vi "Configure Trigger Select.vi"(4 "Hold Type (0: TI)":u16(ring) items=["TI", "TL", "EV", "PS", "PL", "IS", "IL", "P2", "I2", "OFF"], 5 "QL (1: Channel 2)":u16(ring)=1 items=["Channel 1", "Channel 2", "Channel 3", "Channel 4", "Ext", "Ext10", "Line", "Pattern"], 6 "Trigger type":u16(ring) items=["Edge", "Dropout", "Glitch", "Interval", "Std", "Sng", "State Qualify", "Edge Qualify", "Width", "Logic", "Runt", "Slew"], 7 "Trigger Source (0: Channel 1)":u16(ring) items=["Channel 1", "Channel 2", "Channel 3", "Channel 4", "Ext", "Ext10", "Line", "Pattern"], 8 "error in (no error)":errorcluster, 9 "Hold Value 2 (6 ns)":dbl=6e-09, 10 "Hold Value 1 (4 ns)":dbl=4e-09, 11 "VISA resource name":refnum<visa-resource-name>) -> (0 "error out":errorcluster, 3 "VISA resource name out":refnum<visa-resource-name>)   [LabVIEW 2013, in "LeCroy Wave Series.lvlib"]
doc: "Selects the condition that will trigger the acquisition of waveforms. Depending on the trigger type, additional parameters may need to be specified."
uses:
  <instrlib>/LeCroy Wave Series/LeCroy Wave Series.lvlib
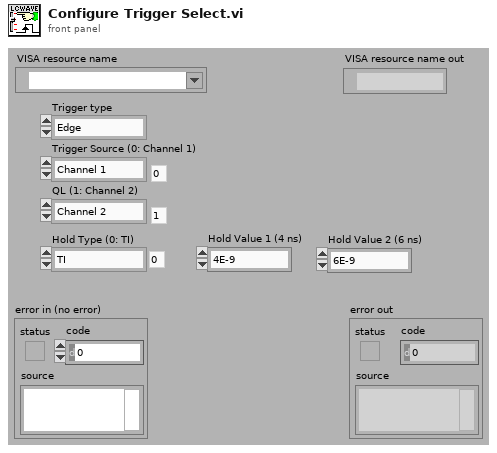
[diagram p1: front panel]
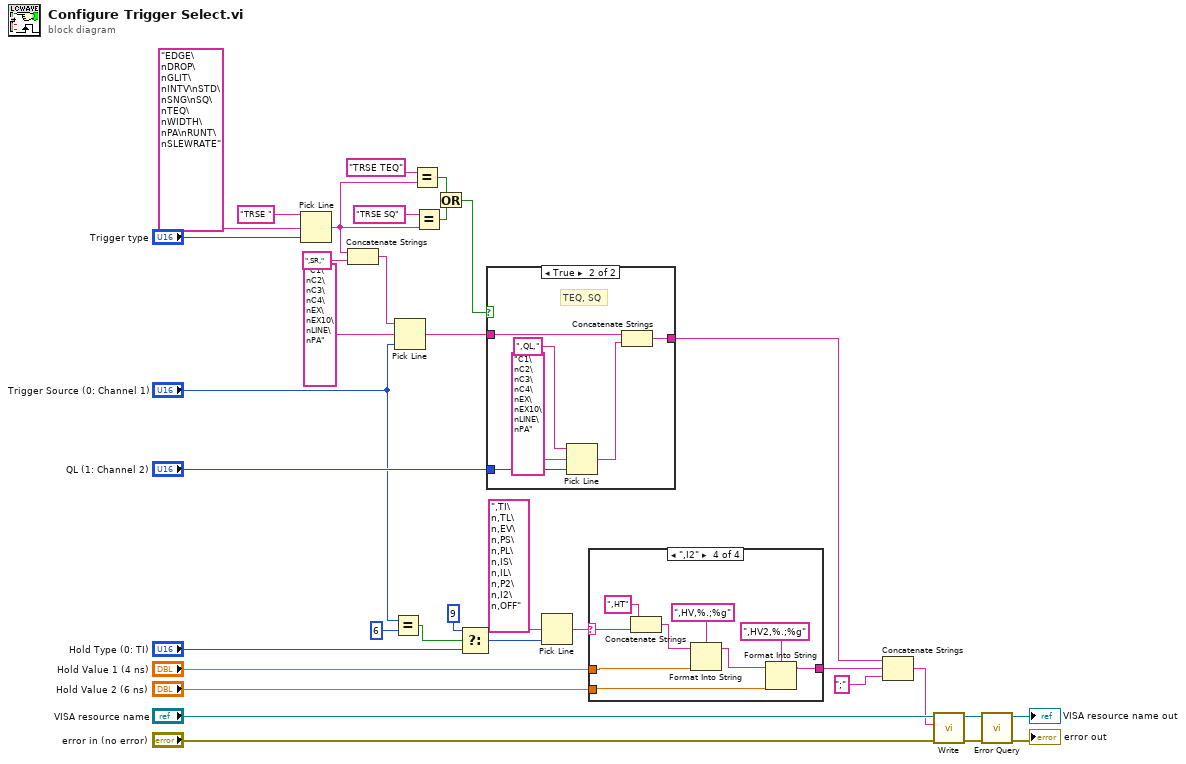
[diagram p0: block diagram]
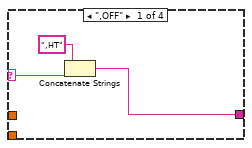
[diagram p2: hidden frame]
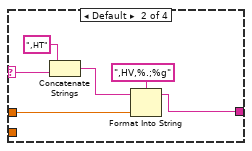
[diagram p3: hidden frame]
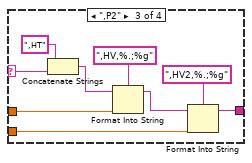
[diagram p4: hidden frame]
diagram:
  n1 = Pick Line(string ("")="TRSE ", multi-line string="EDGE\nDROP\nGLIT\nINTV\nSTD\nSNG\nSQ\nTEQ\nWIDTH\nPA\nRUNT\nSLEWRATE", line index="Trigger type") -> (output string=w25:string)
  n2 = Concatenate Strings(w25, ",SR,") -> (w27:string)
  n3 = Equal?(x="Trigger Source (0: Channel 1)", y=u16 6) -> (x = y?=w10:bool)
  n4 = Pick Line(string ("")=w27, multi-line string="C1\nC2\nC3\nC4\nEX\nEX10\nLINE\nPA", line index="Trigger Source (0: Channel 1)") -> (output string=w20:string)
  n5 = Equal?(x="TRSE TEQ", y=w25) -> (x = y?=w23:bool)
  n6 = Equal?(x="TRSE SQ", y=w25) -> (x = y?=w22:bool)
  n7 = Or(x=w23, y=w22) -> (x .or. y?=w21:bool)
  n8 = Select(t=u16 9, s=w10, f="Hold Type (0: TI)") -> (s? t:f=w5:u16)
  n9 = case shown="True" w21 {
    tunnel: w20 -> [w35 w37]
    tunnel: [w35 w38] -> w14
    tunnel: "QL (1: Channel 2)" -> [_ w40]
    frame False {
      # "EDGE, DROP, GLIT, INTV"
    }
    frame True {
      # "TEQ, SQ"
      n10 = Pick Line(string ("")=",QL,", multi-line string="C1\nC2\nC3\nC4\nEX\nEX10\nLINE\nPA", line index=w40) -> (output string=w36:string)
      n11 = Concatenate Strings(w37, w36) -> (w38:string)
    }
  }
  n12 = Pick Line(multi-line string=",TI\n,TL\n,EV\n,PS\n,PL\n,IS\n,IL\n,P2\n,I2\n,OFF", line index=w5) -> (output string=w17:string)  [unwired: 1 in]
  n13 = case shown="\",I2\"" w17 {
    selector: w17 -> [w43 w46 w52 w61]
    tunnel: "Hold Value 1 (4 ns)" -> [_ w49 w59 w65]
    tunnel: "Hold Value 2 (6 ns)" -> [_ _ w56 w64]
    tunnel: [w42 w48 w54 w63] -> w13
    frame ",OFF" {
      n14 = Concatenate Strings(",HT", w43) -> (w42:string)
    }
    frame Default {
      n15 = Concatenate Strings(",HT", w46) -> (w45:string)
      n16 = Format Into String(format string=",HV,%.;%g", initial string=w45, w49) -> (resulting string=w48:string)  [unwired: 1 in, 1 out]
    }
    frame ",P2" {
      n17 = Concatenate Strings(",HT", w52) -> (w51:string)
      n18 = Format Into String(format string=",HV,%.;%g", initial string=w51, w59) -> (resulting string=w55:string)  [unwired: 1 in, 1 out]
      n19 = Format Into String(format string=",HV2,%.;%g", initial string=w55, w56) -> (resulting string=w54:string)  [unwired: 1 in, 1 out]
    }
    frame ",I2" {
      n20 = Concatenate Strings(",HT", w61) -> (w60:string)
      n21 = Format Into String(format string=",HV,%.;%g", initial string=w60, w65) -> (resulting string=w66:string)  [unwired: 1 in, 1 out]
      n22 = Format Into String(format string=",HV2,%.;%g", initial string=w66, w64) -> (resulting string=w63:string)  [unwired: 1 in, 1 out]
    }
  }
  n23 = Concatenate Strings(w14, w13, ";" ("string")) -> (w11:string)
  n24 = call <instrlib>:"Write.vi"("error in (no error)"="error in (no error)", "Write Buffer"=w11, "VISA resource name"="VISA resource name") -> ("error out"=w3:errorcluster, "VISA resource name out"=w4:refnum<visa-resource-name>)  [unwired: 6 in, 1 out]
  n25 = call <instrlib>:"Error Query.vi"("error in (no error)"=w3, "VISA resource name"=w4) -> ("error out"=→"error out":errorcluster, "VISA resource name out"=→"VISA resource name out":refnum<visa-resource-name>)  [unwired: 6 in, 2 out]
